vi "Launch Data Logger.vi"(8 "error in":errorcluster, 11 "Series Actor in":refnum<class "Series Actor.lvclass">) -> (0 "error out":errorcluster, 3 "Series Actor out":refnum<class "Series Actor.lvclass">)   [LabVIEW 2023, in "Series Actor.lvlib" / "Series Actor.lvclass"]
uses:
  Series Actor.lvclass
  C:/Program Files/National Instruments/LabVIEW 2023/vi.lib/MGI/Panel Manager/Panel Actor/Panel Actor/Panel Actor.lvclass
  Data Logger Actor/Data Logger Actor/Data Logger Actor/Data Logger Actor.lvclass
  Data Sink/IData Sink/IData Sink.lvclass
  Series Actor.lvclass/Series Actor.ctl
  Data Logger Actor/Data Logger Actor/Data Logger Actor/Data Logger Actor.lvclass/Data Logger Actor.ctl
  bbf2da34-f051-41c2-8a30-0667e349fa53.vi
  101dfa38-28b4-4546-847f-5d9f51ff918a.vi
  bbf2da34-f051-41c2-8a30-0667e349fa53.vi/a4169a97-72fc-4003-a778-603cf20cafa0.vi
  <vilib>/JDP Science/JSONtext/Find Item.vi
  <vilib>/JDP Science/JSONtext/Next JSON Value.vi
  <vilib>/JDP Science/JSONtext/String Subset.vi
  <vilib>/JDP Science/JSONtext/Parsing/Advance past next JSON Value (inlined COPY).vi
  <vilib>/JDP Science/JSONtext/Parsing/Advance past whitespace.vi
  <vilib>/JDP Science/JSONtext/Parsing/Advance past String.vi
  <vilib>/JDP Science/JSONtext/Parsing/Advance past Number.vi
  <vilib>/JDP Science/JSONtext/Parsing/Advance past Line Ending.vi
  <vilib>/MGI/Panel Manager/Panel/Panel/Window/Window.lvclass
  C:/Program Files/National Instruments/LabVIEW 2023/vi.lib/MGI/Panel Manager/Panel/Panel/Panel.lvclass
  <vilib>/JDP Science/JSONtext/Parsing/Parse Full Path or Item Name.vi
  <vilib>/JDP Science/JSONtext/Parsing/Advance past Array.vi
  <vilib>/JDP Science/JSONtext/Parsing/Advance past Object.vi
  <vilib>/JDP Science/JSONtext/support/Error Cluster From Code.vi
  <vilib>/JDP Science/JSONtext/Offset/Find Item Locations by Path.vi
  <vilib>/JDP Science/JSONtext/JSON text to Variant.vi
  <vilib>/Utility/error.llb/Error Cluster From Error Code.vi
  <vilib>/MGI/Panel Manager/Panel/Panel/Window/Window.vi
  <vilib>/JDP Science/JSONtext/LVClass Serializer/JSONtext LVClass Serializer.lvclass
  <vilib>/MGI/Panel Manager/Panel Actor/Panel Actor/Panel Actor.lvclass
  <vilib>/MGI/Panel Manager/Panel/Panel.lvlib
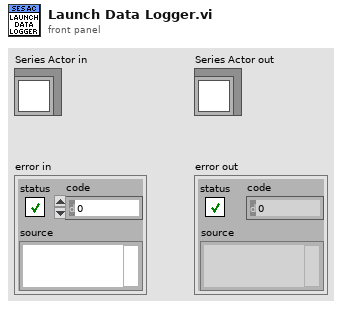
[diagram p1: front panel]
types:
  T1 = cluster{"Class":string, "<JSON>Data Sink":string}
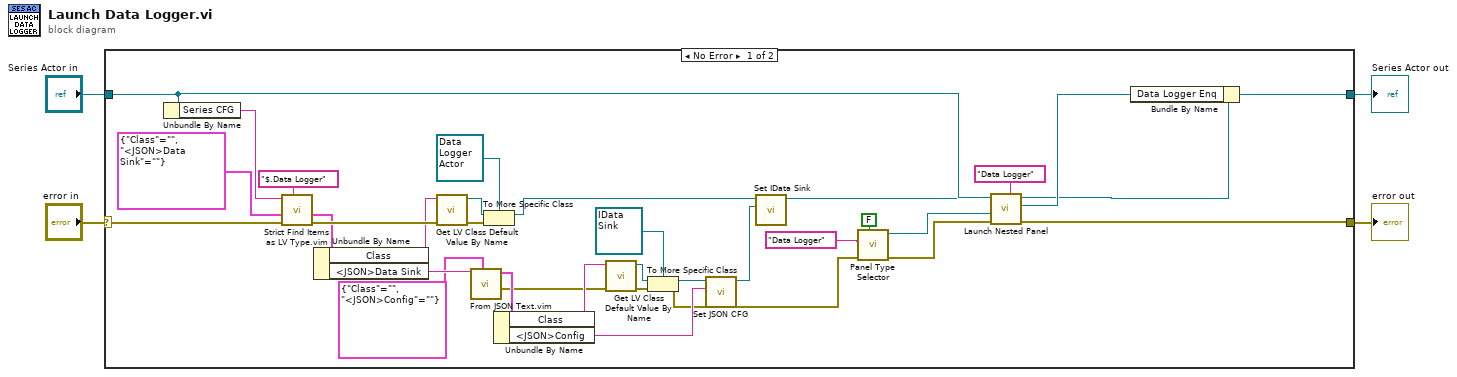
[diagram p0: block diagram]
diagram:
  n1 = case shown="No Error" "error in" {
    selector: "error in" -> [w38 w40]
    tunnel: [w33 w40] -> w3
    tunnel: [w35 w39] -> w1
    tunnel: "Series Actor in" -> [w34 w39]
    frame No Error {
      n2 = Unbundle By Name(w34) -> ("Series CFG"=w37:string)
      n3 = call "Strict Find Items as LV Type.vim"("$Path or Item Name"="$.Data Logger", "error in"=w38, "Data Type and Default Value"=T1 {"Class"="", "<JSON>Data Sink"=""}, "<JSON>"=w37) -> ("error out"=w36:errorcluster, "Data out"=w19:T1)  [unwired: 5 in, 1 out]
      n4 = Unbundle By Name(w19) -> ("Class"=w18:string, "<JSON>Data Sink"=w16:string)
      n5 = call <vilib>:"Get LV Class Default Value By Name.vi"("error in (no error)"=w36, "class name"=w18) -> ("error out"=w32:errorcluster, "object"=w31:refnum<class>)  [unwired: 8 in]
      n6 = call "From JSON Text.vim"("Data Type and Default Value"=cluster{"Class":string, "<JSON>Config":string} {"Class"="", "<JSON>Config"=""}, "JSON"=w16) -> ("error out"=w12:errorcluster, "Data out"=w14:cluster{"Class":string, "<JSON>Config":string})  [unwired: 8 in]
      n7 = To More Specific Class(target class=refnum<class "Data Logger Actor.lvclass"> refnum ("Data Logger Actor.lvlib:Data Logger Actor.lvclass"), reference=w31, error in=w32) -> (specific class reference=w27:refnum<class "Data Logger Actor.lvclass">)  [unwired: 1 out]
      n8 = Unbundle By Name(w14) -> ("Class"=w13:string, "<JSON>Config"=w8:string)
      n9 = call <vilib>:"Get LV Class Default Value By Name.vi"("error in (no error)"=w12, "class name"=w13) -> ("error out"=w10:errorcluster, "object"=w11:refnum<class>)  [unwired: 8 in]
      n10 = To More Specific Class(target class=refnum<class "IData Sink.lvclass"> refnum ("IData Sink.lvclass"), reference=w11, error in=w10) -> (specific class reference=w6:refnum<class "IData Sink.lvclass">, error out=w5:errorcluster)
      n11 = call-dynamic "Set JSON CFG.vi"("<JSON>Data SInk CFG"=w8, "IData Sink in"=w6) -> ("IData Sink out"=w7:refnum<class "IData Sink.lvclass">)  [unwired: 9 in]
      n12 = call "Set IData Sink.vi"("IData Sink"=w7, "Data Logger Actor in"=w27) -> ("Data Logger Actor out"=w17:refnum<class "Data Logger Actor.lvclass">)  [unwired: 9 in]
      n13 = call-poly <vilib>:"Panel Type Selector.vi"("Autoshow? (T)"=FALSE, "error in (no error)"=w5, "Default Title"="Data Logger") -> ("error out"=w25:errorcluster, "Window out"=w23:refnum<class "Window.lvclass">)  [unwired: 7 in]
      n14 = call <vilib>:"Launch Nested Panel.vi"("Debug Alias"="Data Logger", "error in (no error)"=w25, "Panel"=w23, "Nested Panel Actor"=w17, "Panel Actor in"=w34) -> ("error out"=w33:errorcluster, "Nested Actor's Enqueuer"=w30:refnum<class "Message Enqueuer.lvclass">, "Panel Actor out"=w29:refnum<class "Series Actor.lvclass">)  [unwired: 3 in, 1 out]
      n15 = Bundle By Name(cluster=w29, "Data Logger Enq"=w30) -> (w35:refnum<class "Series Actor.lvclass">)
    }
    frame Error {
    }
  }
  "error out" <- w3
  "Series Actor out" <- w1
